vi "Test 1.vi"   [LabVIEW 2016]
types:
  T1 = typedef "LVHSConnector.ctl" = refnum<class "BrickReference.lvclass">
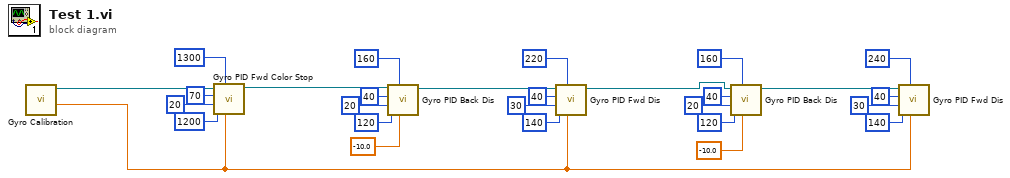
[diagram p0: block diagram]
diagram:
  n1 = call "Gyro Calibration.vi"() -> ("Degrees"=w3:sgl, "NXT/EV3"=w28:T1)  [unwired: 7 in, 1 out]
  n2 = call "Gyro PID Fwd Color Stop.vi"("Target angle"=w3, "Threshold to Color"=1300 ("Threshold to stop"), "Threshold to slow"=1200, "Min. speed"=20, "Max. speed"=70, "EV3 in"=w28) -> ("EV3 out"=w23:T1)  [unwired: 5 in]
  n3 = call "Gyro PID Back Dis.vi"("Target angle"=sgl -10.0, "Threshold to stop"=160, "Threshold to slow"=120, "Min. speed"=20, "Max. speed"=40, "EV3 in"=w23) -> ("EV3 out"=w18:T1)  [unwired: 5 in]
  n4 = call "Gyro PID Fwd Dis.vi"("Target angle"=w3, "Threshold to stop"=220, "Threshold to slow"=140, "Min. speed"=30, "Max. speed"=40, "EV3 in"=w18) -> ("EV3 out"=w4:T1)  [unwired: 5 in]
  n5 = call "Gyro PID Back Dis.vi"("Target angle"=sgl -10.0, "Threshold to stop"=160, "Threshold to slow"=120, "Min. speed"=20, "Max. speed"=40, "EV3 in"=w4) -> ("EV3 out"=w9:T1)  [unwired: 5 in]
  n6 = call "Gyro PID Fwd Dis.vi"("Target angle"=w3, "Threshold to stop"=240, "Threshold to slow"=140, "Min. speed"=30, "Max. speed"=40, "EV3 in"=w9) -> ()  [unwired: 5 in, 1 out]
